vi "Send Direct Unlock Publication.vi"(6 "Publisher ID":string, 7 "Message Priority (Normal)":T1=enum."Normal", 8 "error in (no error)":errorcluster, 9 "Datum Type":variant, 10 "Datum Name":string, 11 "Mediator Enqeuer":refnum<class "Message Enqueuer.lvclass">) -> (0 "error out":errorcluster, 3 "Mediator Enqueuer out":refnum<class "Message Enqueuer.lvclass">)   [LabVIEW 2020, in "MVA Framework.lvlib" / "IMediator.lvlib" / "Unlock Publication Msg.lvclass"]
doc: "此VI直接向中介发送消息（例如ViewModel可能希望发布通用系统数据（如状态）供视图观察的情况）。只有控制器应该有一个到中介的直接队列，因此任何非控制器类都不太可能调用这个VI。"
uses:
  Unlock Publication Msg.lvclass
  <vilib>/ActorFramework/Message Enqueuer/Message Enqueuer.lvclass
  <vilib>/ActorFramework/Message Enqueuer/Message Priority.ctl
  C:/Program Files/National Instruments/LabVIEW 2020/vi.lib/ActorFramework/Message/Message.lvclass
  Unlock Publication Msg.lvclass/Unlock Publication Msg.ctl
  <vilib>/ActorFramework/Message Enqueuer/Message Enqueuer.lvclass/Message Enqueuer.ctl
  <vilib>/ActorFramework/Message Priority Queue/Priority Enqueue.vi
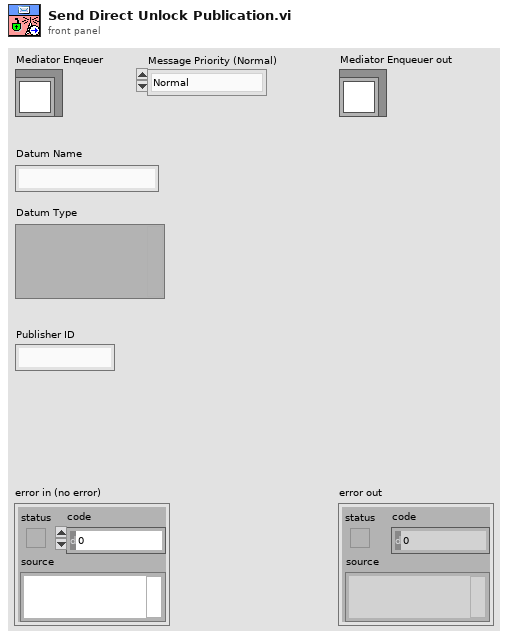
[diagram p1: front panel]
types:
  T1 = typedef "Actor Framework.lvlib/Message Enqueuer.lvclass/Message Priority.ctl" = enum16{"Low", "Normal", "High"}
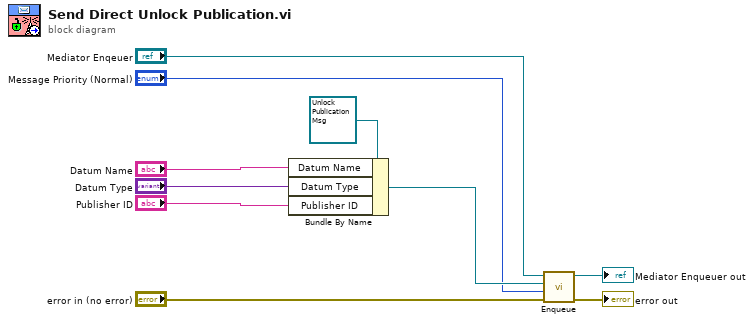
[diagram p0: block diagram]
diagram:
  n1 = Bundle By Name(cluster=refnum<class "Unlock Publication Msg.lvclass"> refnum ("Publish Message"), "Datum Name"="Datum Name", "Datum Type"="Datum Type", "Publisher ID"="Publisher ID") -> (w5:refnum<class "Unlock Publication Msg.lvclass">)
  n2 = call <vilib>:"Enqueue.vi"("error in (no error)"="error in (no error)", "Message Priority (Normal)"="Message Priority (Normal)", "Message"=w5, "Message Enqueuer in"="Mediator Enqeuer") -> ("error out"=→"error out":errorcluster, "Message Enqueuer in"=→"Mediator Enqueuer out":refnum<class "Message Enqueuer.lvclass">)  [unwired: 6 in]
